vi "Check.vi"(8 "error in (no error)":errorcluster, 10 "Encoded string":string, 11 "Encoding in":refnum<class "CConfig UTF-8-BOM Encoding.lvclass">) -> (0 "error out":errorcluster, 1 "Match?":bool, 2 "Encoded string":string, 3 "Encoding out":refnum<class "CConfig UTF-8-BOM Encoding.lvclass">)   [LabVIEW 2013, in "CConfig UTF-8-BOM Encoding.lvclass"]
doc: "Copyright 2018, Carya Automatisering, Wiebe Walstra."
uses:
  CConfig UTF-8-BOM Encoding.lvclass
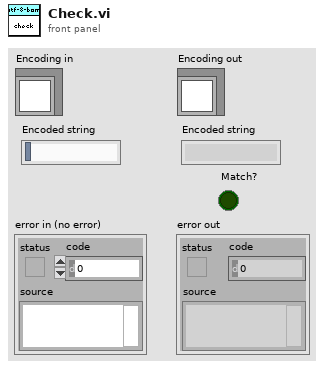
[diagram p1: front panel]
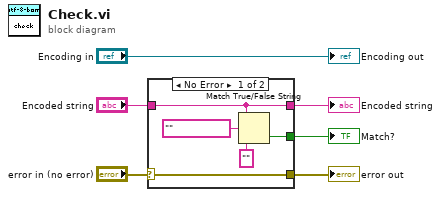
[diagram p0: block diagram]
diagram:
  n1 = case shown="No Error" "error in (no error)" {
    selector: "error in (no error)" -> [w11 w12]
    tunnel: [w11 w12] -> w4
    tunnel: "Encoded string" -> [w7 w13]
    tunnel: [w7 w13] -> w2
    tunnel: [w8 _] -> w1
    frame No Error {
      n2 = Match True/False String(2:"" ("false string"), 3:"﻿" ("true string"), 4:w7) -> (0:w8:bool)  [unwired: 1 out]
    }
    frame Error {
    }
  }
  "error out" <- w4
  "Encoded string" <- w2
  "Match?" <- w1
  "Encoding out" <- "Encoding in"
